vi "DAQmx.44xx.Get Export Triggers.vi"(8 "error in (no error)":errorcluster, 10 "master task in":refnum<k21>, 11 "task in":refnum<k21>) -> (0 "error out":errorcluster, 3 "task out":refnum<k21>)   [LabVIEW 2019, in "DAQmx.lvclass"]
uses:
  DAQmx.lvclass
  <resource>/objmgr/daqmx.rc
  <vilib>/DAQmx/configure/trigger.llb/DAQmx Start Trigger (Digital Edge).vi
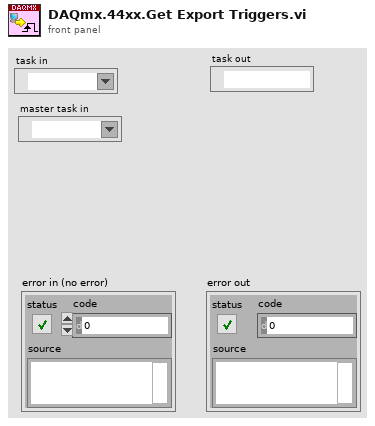
[diagram p1: front panel]
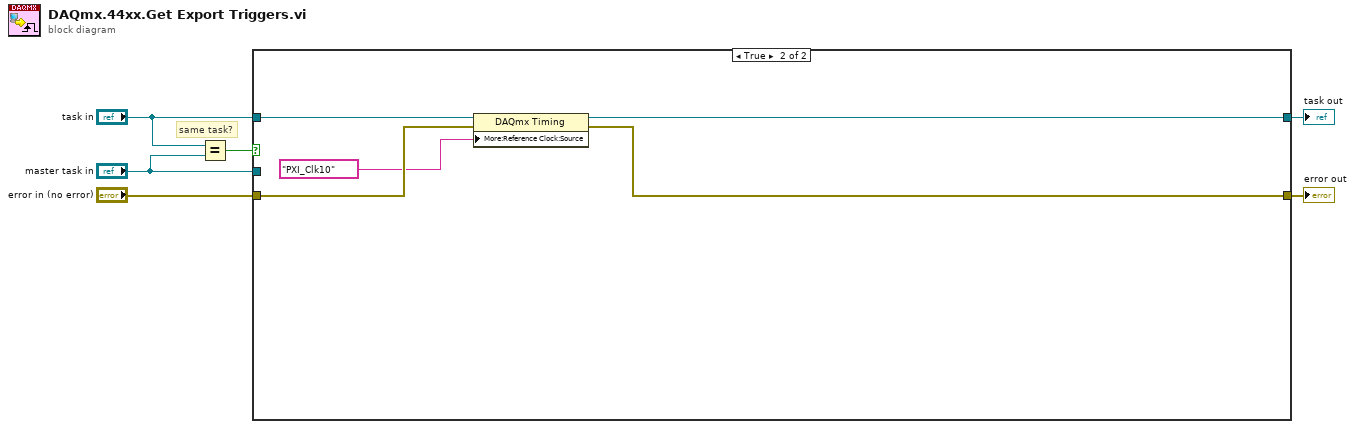
[diagram p0: block diagram]
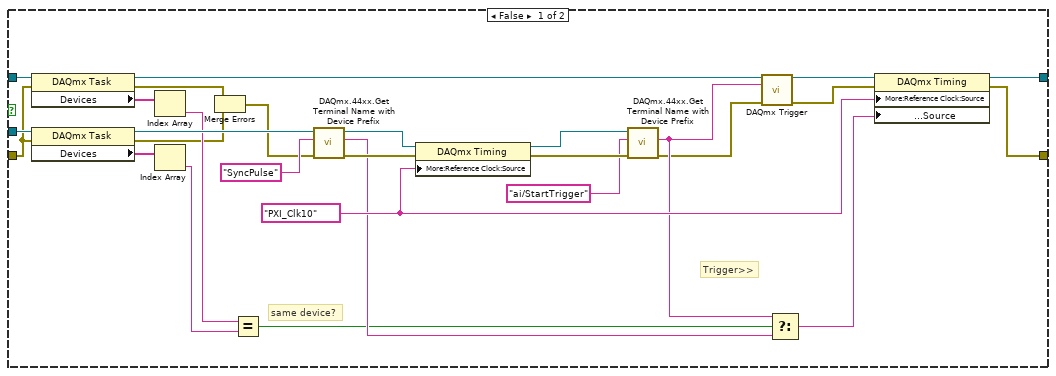
[diagram p2: hidden frame]
diagram:
  # "same task?"
  n1 = Equal?(x="task in", y="master task in") -> (x = y?=w1:bool)
  n2 = case shown="True" w1 {
    tunnel: "error in (no error)" -> [w12 w38]
    tunnel: [w24 w37] -> w5
    tunnel: [w23 w36] -> w4
    tunnel: "master task in" -> [w16 _]
    tunnel: "task in" -> [w14 w39]
    frame False {
      w29 = tag "PXI_Clk10" ("RefClk.Src")
      # "same device?"
      # "Trigger>>"
      n3 = property class="DAQmx Task"(reference=w14, error in=w12) -> (reference out=w15:refnum<k21>, error out=w9:errorcluster, "Devices"=w30:tag[])
      n4 = property class="DAQmx Task"(reference=w16, error in=w12) -> (reference out=w17:refnum<k21>, error out=w8:errorcluster, "Devices"=w13:tag[])
      n5 = Index Array(array=w30) -> (element=w11:tag)  [unwired: 1 in]
      n6 = Index Array(array=w13) -> (element=w10:tag)  [unwired: 1 in]
      n7 = Merge Errors(w9, w8) -> (w7:errorcluster)
      n8 = Equal?(x=w11, y=w10) -> (x = y?=w26:bool)
      n9 = call "DAQmx.44xx.Get Terminal Name with Device Prefix.vi"("error in (no error)"=w7, "Local Terminal Name"="SyncPulse", "task"=w17) -> ("error out"=w33:errorcluster, "Terminal Name with Device Prefix"=w27:tag, "task out"=w19:refnum<k21>)  [unwired: 6 in]
      n10 = property class="DAQmx Timing"(reference=w19, error in=w33, "More:Reference Clock:Source"=w29) -> (reference out=w22:refnum<k21>, error out=w34:errorcluster)
      n11 = call "DAQmx.44xx.Get Terminal Name with Device Prefix.vi"("error in (no error)"=w34, "Local Terminal Name"="ai/StartTrigger", "task"=w22) -> ("error out"=w25:errorcluster, "Terminal Name with Device Prefix"=w28:tag)  [unwired: 6 in, 1 out]
      n12 = call-poly <vilib>:"DAQmx Trigger.vi"("task/channels in"=w15, "source"=w28, "error in"=w25) -> ("task out"=w21:refnum<k21>, "error out"=w20:errorcluster)  [unwired: 11 in]
      n13 = Select(t=w28, s=w26, f=w27) -> (s? t:f=w31:tag)
      n14 = property class="DAQmx Timing"(reference=w21, error in=w20, "More:Reference Clock:Source"=w29, "More:Synchronization Pulse:Source"=w31) -> (reference out=w24:refnum<k21>, error out=w23:errorcluster)
    }
    frame True {
      n15 = property class="DAQmx Timing"(reference=w39, error in=w38, "More:Reference Clock:Source"=tag "PXI_Clk10" ("RefClk.Src")) -> (reference out=w37:refnum<k21>, error out=w36:errorcluster)
    }
  }
  "error out" <- w4
  "task out" <- w5
